vi "Connect_SignatureIn_Signal.vi"(4 "Relay Signal Signature":string, 6 "Relay Object":refnum<class "LQObject.lvclass">, 8 "Error In":errorcluster, 10 "Source Signal Signature":string, 11 "Sender In":refnum<class "LQObject.lvclass">) -> (0 "Error Out":errorcluster, 3 "Sender Out":refnum<class "LQObject.lvclass">)   [LabVIEW 2014, in "LQ Core.lvlib" / "LQCoreEngine.lvclass"]
uses:
  LQCoreEngine.lvclass
  LQObject/LQObject.lvclass
  LQIdentity/LQIdentity.lvclass/LQIdentity.ctl
  LQIdentity/LQIdentity.lvclass
  LQ Core.lvlib
panel:
  # "Copyright (c) 2016 Sze Howe Koh\n\nThis Source Code Form is subject to the terms of the Mozilla Public\nLicense, v. 2.0. If a copy of the MPL was not distributed with this\nfile, You can obtain one at http://mozilla.org/MPL/2.0/."
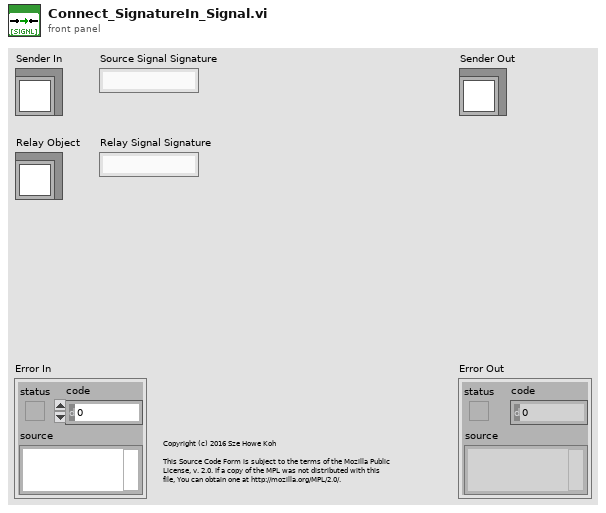
[diagram p1: front panel]
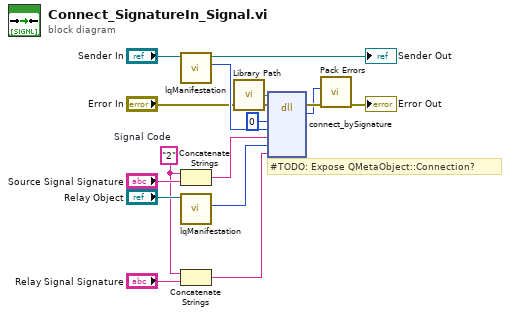
[diagram p0: block diagram]
diagram:
  w1 = "2"  # Signal Code
  # "#TODO: Expose QMetaObject::Connection?"
  n1 = call "lqManifestation.vi"("LQIdentity in"="Sender In") -> ("Manifestation"=w11:u64, "LQIdentity out"=→"Sender Out":refnum<class "LQObject.lvclass">)  [unwired: 9 in]
  n2 = Concatenate Strings(w1, "Source Signal Signature") -> (w6:string)
  n3 = call "lqManifestation.vi"("LQIdentity in"="Relay Object") -> ("Manifestation"=w12:u64)  [unwired: 9 in, 1 out]
  n4 = Concatenate Strings(w1, "Relay Signal Signature") -> (w7:string)
  n5 = call "Library Path.vi"() -> ("Library Path"=w15:path)
  n6 = dll-call lib="?" fn="connect_bySignature"(path in=w15, error in="Error In", "_retVal"=u64 0, "sender"=w11, "encodedSignal"=w6, "receiver"=w12, "encodedMethod"=w7) -> (error out=w5:errorcluster, "errorCode"=w4:i32)  [unwired: 6 in, 1 out]
  n7 = call "Pack Errors.vi"("Error In"=w5, "Error Code"=w4) -> ("Error Out"=→"Error Out":errorcluster)  [unwired: 9 in]
